vi "Test_ReadValue_NeverWritten_StructureTimeout.vi"(8 "error in (no error)":errorcluster, 11 "TestCase in":refnum<class "TestEventTransport.lvclass">) -> (0 "error out":errorcluster, 3 "TestCase out":refnum<class "TestEventTransport.lvclass">)   [LabVIEW 2017, in "TestEventTransport.lvclass"]
uses:
  TestEventTransport.lvclass
  Source/Concrete/EventTransport/EventTransport.lvclass/EventTransport.ctl
  Source/Concrete/EventTransport/EventTransport.lvclass
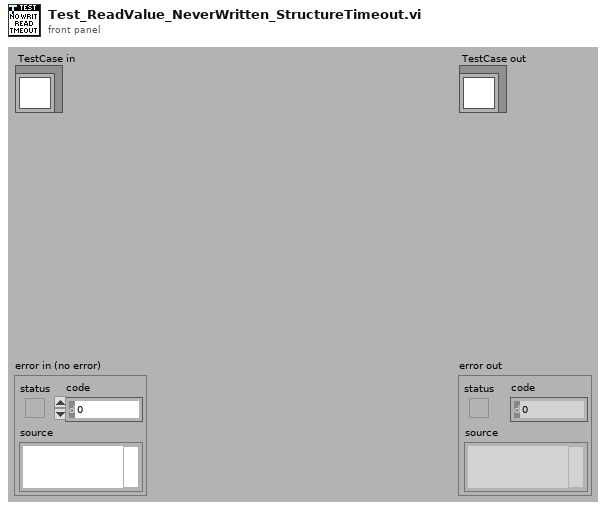
[diagram p1: front panel]
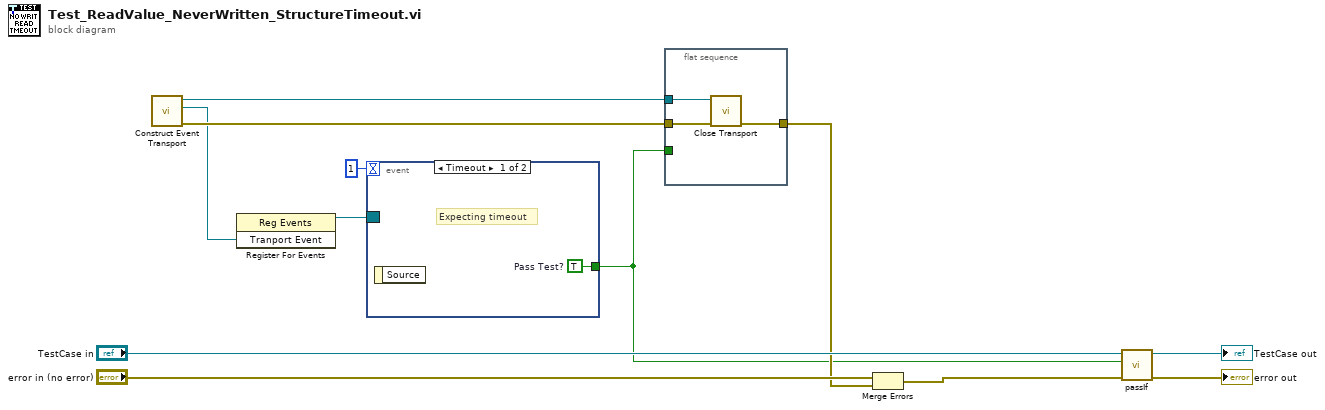
[diagram p0: block diagram]
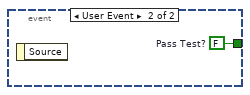
[diagram p2: hidden frame]
diagram:
  n1 = call "Construct Event Transport.vi"() -> ("error out"=w7:errorcluster, "Tranport Event"=w4:refnum<user-event>, "EventTransport"=w5:refnum<class "EventTransport.lvclass">)  [unwired: 9 in]
  n2 = register-events(w4) -> (reference out=w3:refnum<event-registration>)  [unwired: 2 in, 1 out]
  n3 = event shown="[0] Timeout" {
    selector: w3 -> [_ _]
    dyn-events: _ -> [_ _]
    timeout: 1 -> [_ _]
    tunnel: [w13 w14] -> w1
    event Timeout {
      w13 = TRUE  # Pass Test?
      # "Expecting timeout"
      n4 = event-data() -> ()  [unwired: 1 in, 1 out]
    }
    event User Event {
      w14 = FALSE  # Pass Test?
      n5 = event-data() -> ()  [unwired: 1 in, 1 out]
    }
  }
  n6 = flat-sequence {
    tunnel: w7 -> [w17]
    tunnel: [w16] -> w6
    tunnel: w5 -> [w15]
    tunnel: w1 -> [_]
    frame #0 {
      n7 = call-dynamic "Close Transport.vi"("error in (no error)"=w17, "EventTransport"=w15) -> ("error out"=w16:errorcluster)  [unwired: 9 in]
    }
  }
  n8 = Merge Errors("error in (no error)", w6) -> (w8:errorcluster)
  n9 = call-dynamic "passIf.vi"("error in (no error)"=w8, "pass"=w1, "TestCase in"="TestCase in") -> ("error out"=→"error out":errorcluster, "TestCase out"=→"TestCase out":refnum<class "TestEventTransport.lvclass">)  [unwired: 7 in]
